vi "Get Last Item From Node Path.vi"(11 "Name":string) -> (2 "Last Item":string, 3 "First Items":string[](array[string]))   [LabVIEW 2019, in "Simple SysDef API.lvlib"]
uses:
  <userlib>/SimpleSysDef/Simple SysDef API.lvlib
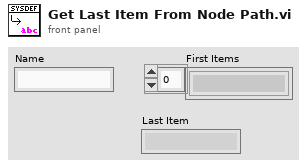
[diagram p1: front panel]
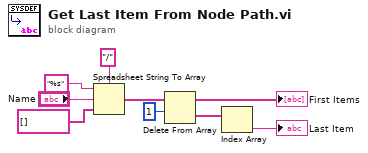
[diagram p0: block diagram]
diagram:
  n1 = Spreadsheet String To Array(delimiter (Tab)="/", format string="%s", spreadsheet string="Name", array type (2D Dbl)=string[] []) -> (array=w5:string[])
  n2 = Delete From Array(array=w5, length=1) -> (deleted portion=w8:string[], array with subset deleted=→"First Items":string[])  [unwired: 1 in]
  n3 = Index Array(array=w8) -> (element=→"Last Item":string)  [unwired: 1 in]
